vi "normalized points generator.vi"(5 "Symmetric":bool, 6 "Stage Control":T1=enum."XY-Y", 7 "FOV(real)":i32=5, 9 "number of points":i32=5, 10 "maximum":dbl=1.0, 11 "minimum":dbl=-1.0) -> (2 "Adjusted array":dbl[](array[numeric]), 3 "normalised array":dbl[](array[numeric]))   [LabVIEW 2020]
uses:
  TypeDefs/Control Plane.ctl
panel:
  out "Array 2":dbl[](array[numeric])
  out "Array":dbl[](array[numeric])
  out "size(s) 2":i32
  out "size(s)":i32
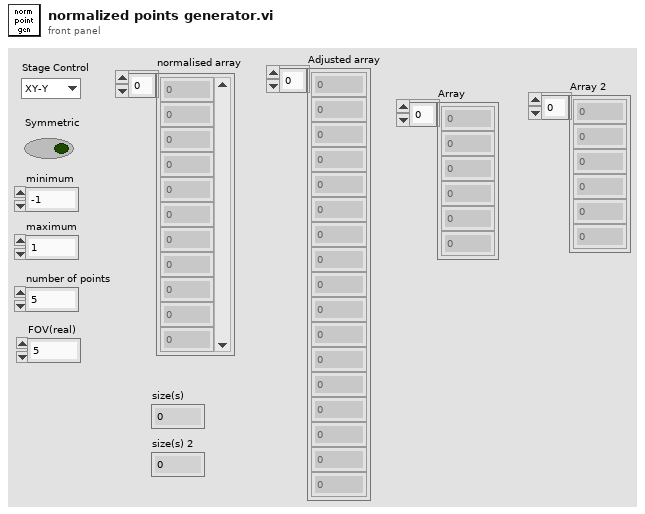
[diagram p1: front panel]
types:
  T1 = typedef "Control Plane.ctl" = enum16{"XY-X", "XY-Y", "Z"}
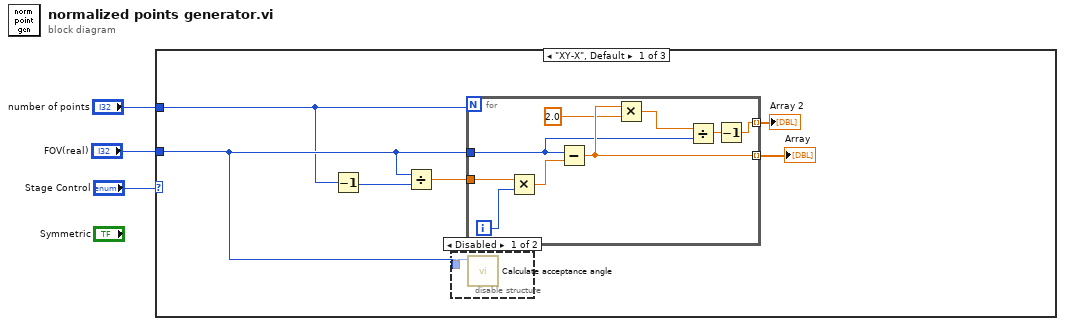
[diagram p0: block diagram]
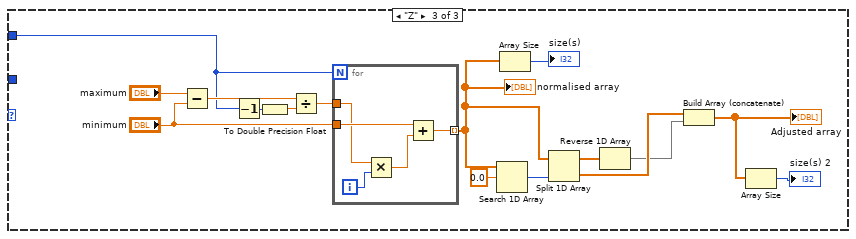
[diagram p4: hidden frame]
diagram:
  n1 = case shown="\"XY-X\", Default" "Stage Control" {
    tunnel: "FOV(real)" -> [w9 _ _]
    tunnel: "number of points" -> [w4 _ w20]
    frame "XY-X", Default {
      n2 = Decrement(x=w4) -> (x-1=w5:i32)
      n3 = Divide(x=w9, y=w5) -> (x/y=w8:dbl)
      n4 = disable-structure shown="Disabled" {
        disable-tunnel: w9 -> [w10 _]
        frame Disabled {
          n5 = call "Calculate acceptance angle.vi"("FOV (true)"=w10) -> ()  [unwired: 9 in, 2 out]
        }
        frame Enabled {
        }
      }
      n6 = for {
        N: w4 -> [_]
        tunnel: w9 -> [w13]
        tunnel: w8 -> [w19]
        tunnel: [w16] -> w7 mode=indexing
        tunnel: [w11] -> w6 mode=indexing
        i -> [w18]
        n7 = Multiply(x=w19, y=w18) -> (x*y=w17:dbl)
        n8 = Subtract(x=w13, y=w17) -> (x-y=w16:dbl)
        n9 = Multiply(x=w16, y=2.0) -> (x*y=w14:dbl)
        n10 = Divide(x=w14, y=w13) -> (x/y=w12:dbl)
        n11 = Decrement(x=w12) -> (x-1=w11:dbl)
      }
      "Array" <- w7
      "Array 2" <- w6
    }
    frame "XY-Y" {
    }
    frame "Z" {
      n12 = Subtract(x="maximum", y="minimum") -> (x-y=w33:dbl)
      n13 = Decrement(x=w20) -> (x-1=w30:i32)
      n14 = To Double Precision Float(number=w30) -> (double precision float=w32:dbl)
      n15 = Divide(x=w33, y=w32) -> (x/y=w31:dbl)
      n16 = for {
        N: w20 -> [_]
        tunnel: "minimum" -> [w40]
        tunnel: w31 -> [w38]
        tunnel: [w36] -> w26 mode=indexing
        i -> [w39]
        n17 = Multiply(x=w38, y=w39) -> (x*y=w37:dbl)
        n18 = Add(x=w40, y=w37) -> (x+y=w36:dbl)
      }
      "normalised array" <- w26
      n19 = Search 1D Array(1D array=w26, element=0.0) -> (index of element=w27:i32)  [unwired: 1 in]
      n20 = Array Size(array=w26) -> (size(s)=→"size(s)":i32)
      n21 = Split 1D Array(array=w26, index=w27) -> (first subarray=w25:dbl[], second subarray=w24:dbl[])
      n22 = Reverse 1D Array(array=w25) -> (reversed array=w23:dbl[])
      n23 = Build Array (concatenate)(w24, w23) -> (w21:dbl[])
      "Adjusted array" <- w21
      n24 = Array Size(array=w21) -> (size(s)=→"size(s) 2":i32)
    }
  }
